vi "ex_PrepareDAQmx.vi"(2 "error in":errorcluster, 3 "task/channels in":refnum<k21>) -> (0 "error out":errorcluster, 1 "task out":refnum<k21>)   [LabVIEW 2017]
uses:
  <resource>/objmgr/daqmx.rc
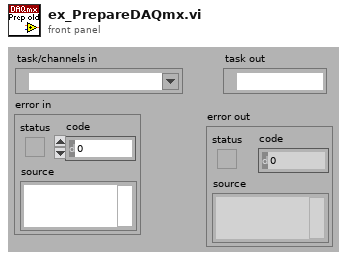
[diagram p1: front panel]
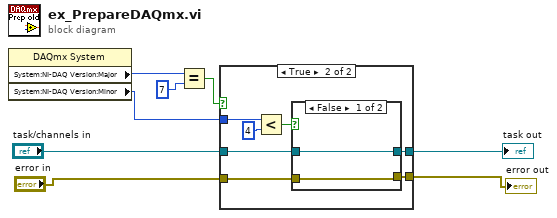
[diagram p0: block diagram]
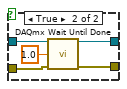
[diagram p3: hidden frame]
diagram:
  n1 = property class="DAQmx System"() -> ("System:NI-DAQ Version:Major"=w7:u32, "System:NI-DAQ Version:Minor"=w8:u32)  [unwired: 2 in, 2 out]
  n2 = Equal?(x=w7, y=u32 7) -> (x = y?=w5:bool)
  n3 = case shown="True" w5 {
    tunnel: w8 -> [_ w16]
    tunnel: "task/channels in" -> [w10 w14]
    tunnel: [w10 w13] -> w3
    tunnel: "error in" -> [w9 w12]
    tunnel: [w9 w11] -> w1
    frame False {
    }
    frame True {
      n4 = Less?(x=w16, y=u32 4) -> (x < y?=w15:bool)
      n5 = case shown="False" w15 {
        tunnel: w14 -> [w19 w24]
        tunnel: [w19 w23] -> w13
        tunnel: w12 -> [w18 w21]
        tunnel: [w18 w20] -> w11
        frame False {
        }
        frame True {
          n6 = call <vilib>:"DAQmx Wait Until Done.vi"("task/channels in"=w24, "timeout (sec)"=1.0, "error in"=w21) -> ("task out"=w23:refnum<k21>, "error out"=w20:errorcluster)  [unwired: 11 in]
        }
      }
    }
  }
  "task out" <- w3
  "error out" <- w1
